vi "Start Synchronization.vi"(8 "error in (no error)":errorcluster, 10 "Interval (ms)":i32, 11 "Application in":refnum<class "Application.lvclass">) -> (0 "error out":errorcluster, 3 "Application out":refnum<class "Application.lvclass">)   [LabVIEW 2015]
uses:
  Hardware/Synchronization Device/Synchronization Device.lvclass
  <vilib>/ActorFramework/Actor/Actor.lvclass
  Application.lvclass
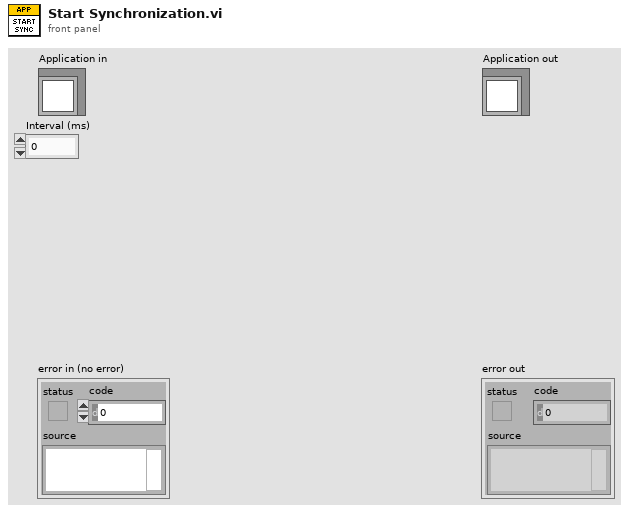
[diagram p1: front panel]
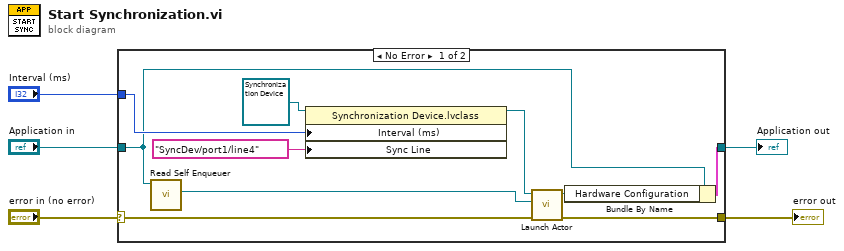
[diagram p0: block diagram]
diagram:
  n1 = case shown="No Error" "error in (no error)" {
    selector: "error in (no error)" -> [w9 w17]
    tunnel: [w8 w17] -> w4
    tunnel: [w15 w16] -> w2
    tunnel: "Application in" -> [w7 w16]
    tunnel: "Interval (ms)" -> [w11 _]
    frame No Error {
      n2 = call <vilib>:"Read Self Enqueuer.vi"("Actor"=w7) -> ("Self Enqueuer"=w6:refnum<class "Message Enqueuer.lvclass">)  [unwired: 10 in]
      n3 = property class="Synchronization Device.lvclass"(reference=refnum<class "Synchronization Device.lvclass"> refnum ("Synchronization Device.lvlib:Synchronization Device.lvclass"), "Interval (ms)"=w11, "Sync Line"=tag "SyncDev/port1/line4" ("lines")) -> (reference out=w13:refnum<class "Synchronization Device.lvclass">)  [unwired: 1 in, 1 out]
      n4 = call <vilib>:"Launch Actor.vi"("error in (no error)"=w9, "Actor-to-Caller Enqueuer"=w6, "Actor"=w13) -> ("error out"=w8:errorcluster, "Caller-To-Actor Enqueuer"=w10:refnum<class "Message Enqueuer.lvclass">)  [unwired: 7 in]
      n5 = Bundle By Name(cluster=w7, "Hardware Configuration"=w10) -> (w15:cluster{})
    }
    frame Error {
    }
  }
  "error out" <- w4
  "Application out" <- w2
